vi "Gradient Power Supply Initializer.vi"(8 "error in":errorcluster, 10 "Gradient Supply Address":string, 11 "Gradient Supply Type":string) -> (0 "error out":errorcluster)   [LabVIEW 2016]
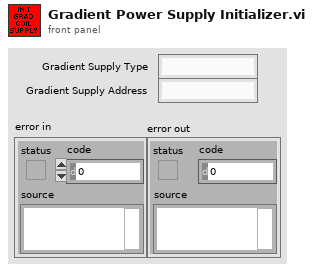
[diagram p1: front panel]
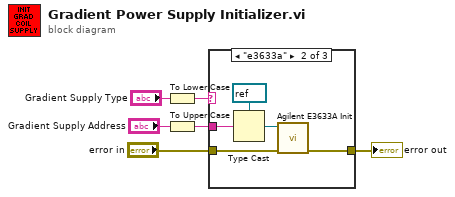
[diagram p0: block diagram]
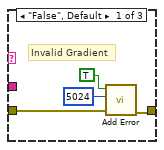
[diagram p2: hidden frame]
diagram:
  n1 = To Lower Case(string="Gradient Supply Type") -> (all lower case string=w5:string)
  n2 = To Upper Case(1:"Gradient Supply Address") -> (0:w2:string)
  n3 = case shown="\"e3633a\"" w5 {
    tunnel: [w9 w14 w16] -> w1
    tunnel: "error in" -> [w10 w15 w16]
    tunnel: w2 -> [_ w13 _]
    frame "False", Default {
      # "Invalid Gradient"
      n4 = call "Add Error.vi"("error in (no error)"=w10, "error code (0)"=5024, "error?"=TRUE) -> ("error out"=w9:errorcluster)  [unwired: 8 in]
    }
    frame "e3633a" {
      n5 = Type Cast(type=refnum<k15> refnum ("resource name"), x=w13) -> (*(type *) &x=w11:refnum<k15>)
      n6 = call "Agilent E3633A Init.vi"("error in (no error)"=w15, "resource name"=w11) -> ("error out"=w14:errorcluster)  [unwired: 6 in, 1 out]
    }
    frame "rri_loadgo" {
    }
  }
  "error out" <- w1
